vi "GetUncertaintyPath.vi"(8 "error in (no error)":errorcluster, 11 "FileName":string) -> (0 "error out":errorcluster, 3 "Path":path)   [LabVIEW 2014]
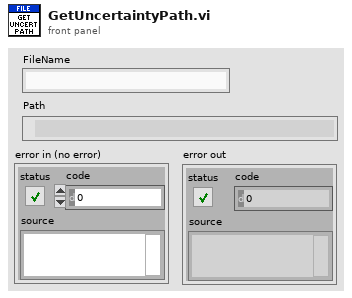
[diagram p1: front panel]
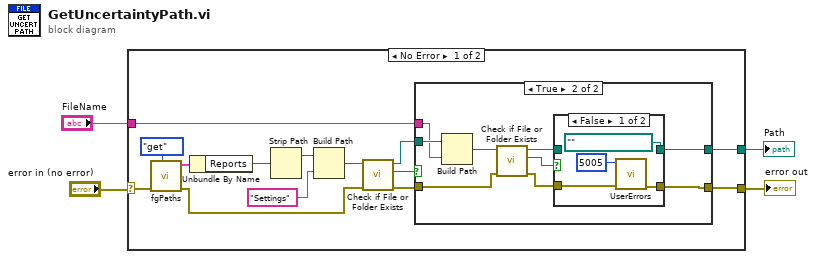
[diagram p0: block diagram]
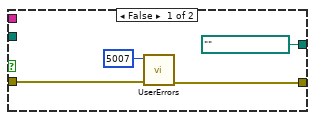
[diagram p2: hidden frame]
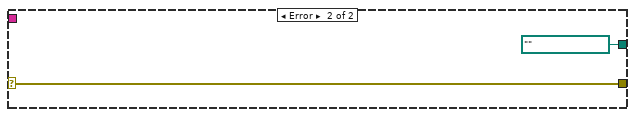
[diagram p4: hidden frame]
diagram:
  n1 = case shown="No Error" "error in (no error)" {
    selector: "error in (no error)" -> [w17 w39]
    tunnel: [w5 w39] -> w3
    tunnel: "FileName" -> [w9 _]
    tunnel: [w6 path "" ("dup path")] -> w1
    frame No Error {
      n2 = call "fgPaths.vi"("cmd"=enum16{"init", "set", "get"}."get", "error in (no error)"=w17) -> ("error out"=w12:errorcluster, "clPaths"=w16:cluster{"Templates":path, "Reports":path})  [unwired: 8 in]
      n3 = Unbundle By Name(w16) -> ("Reports"=w15:path)
      n4 = Strip Path(path=w15) -> (stripped path=w8:path)  [unwired: 1 out]
      n5 = Build Path(base path=w8, name or relative path="Settings") -> (appended path=w13:path)
      n6 = call <vilib>:"Check if File or Folder Exists.vi"("error in (no error)"=w12, "path"=w13) -> ("error out"=w10:errorcluster, "file or folder exists?"=w11:bool, "dup path"=w7:path)  [unwired: 7 in]
      n7 = case shown="True" w11 {
        tunnel: w10 -> [w21 w28]
        tunnel: [w20 w24] -> w5
        tunnel: w9 -> [_ w30]
        tunnel: w7 -> [_ w31]
        tunnel: [path "" ("dup path") w23] -> w6
        frame False {
          n8 = call "UserErrors.vi"("error in (no error)"=w21, "[error code] (0)"=5007) -> ("error out"=w20:errorcluster)  [unwired: 9 in]
        }
        frame True {
          n9 = Build Path(base path=w31, name or relative path=w30) -> (appended path=w29:path)
          n10 = call <vilib>:"Check if File or Folder Exists.vi"("error in (no error)"=w28, "path"=w29) -> ("error out"=w25:errorcluster, "file or folder exists?"=w27:bool, "dup path"=w26:path)  [unwired: 7 in]
          n11 = case shown="False" w27 {
            tunnel: w26 -> [_ w36]
            tunnel: w25 -> [w34 w37]
            tunnel: [w33 w37] -> w24
            tunnel: [path "" ("dup path") w36] -> w23
            frame False {
              n12 = call "UserErrors.vi"("error in (no error)"=w34, "[error code] (0)"=5005) -> ("error out"=w33:errorcluster)  [unwired: 9 in]
            }
            frame True {
            }
          }
        }
      }
    }
    frame Error {
    }
  }
  "error out" <- w3
  "Path" <- w1
